vi "get limits from circle.vi"(8 "Radius":dbl, 10 "Current Location":T1 {"Position"."Position Y" format="%#.3f"; "Position"."Position X" format="%#.3f"}, 11 "Center location":T1 {"Position"."Position Y" format="%#.3f"; "Position"."Position X" format="%#.3f"}) -> (0 "Ymax given x":dbl, 1 "Ymin given x":dbl, 2 "Xmax given y":dbl, 3 "Xmin given y":dbl)   [LabVIEW 2017]
uses:
  location.ctl
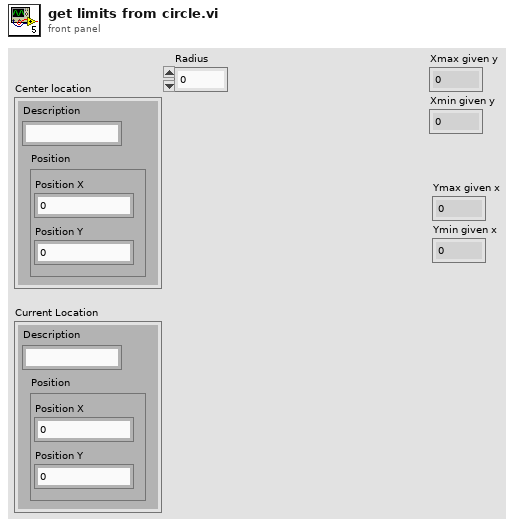
[diagram p1: front panel]
types:
  T1 = typedef "location.ctl" = cluster{"Description":string, "Position":cluster{"Position X":dbl, "Position Y":dbl}}
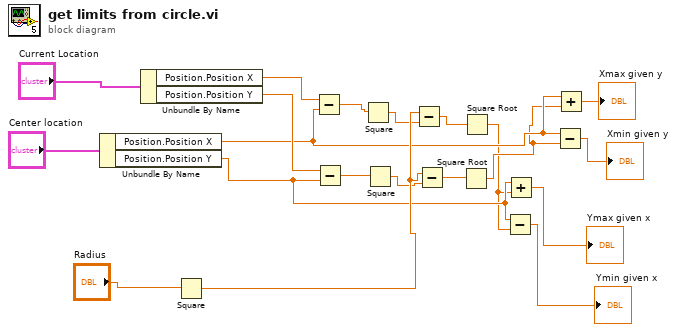
[diagram p0: block diagram]
diagram:
  n1 = Unbundle By Name("Center location") -> ("Position.Position X"=w6:dbl, "Position.Position Y"=w4:dbl)
  n2 = Unbundle By Name("Current Location") -> ("Position.Position X"=w18:dbl, "Position.Position Y"=w17:dbl)
  n3 = Square(x="Radius") -> (x^2=w13:dbl)
  n4 = Subtract(x=w18, y=w6) -> (x-y=w15:dbl)
  n5 = Subtract(x=w17, y=w4) -> (x-y=w14:dbl)
  n6 = Square(x=w15) -> (x^2=w12:dbl)
  n7 = Square(x=w14) -> (x^2=w11:dbl)
  n8 = Subtract(x=w13, y=w12) -> (x-y=w10:dbl)
  n9 = Subtract(x=w13, y=w11) -> (x-y=w9:dbl)
  n10 = Square Root(x=w9) -> (sqrt(x)=w5:dbl)
  n11 = Square Root(x=w10) -> (sqrt(x)=w3:dbl)
  n12 = Subtract(x=w4, y=w3) -> (x-y=→"Ymin given x":dbl)
  n13 = Add(x=w4, y=w3) -> (x+y=→"Ymax given x":dbl)
  n14 = Subtract(x=w6, y=w5) -> (x-y=→"Xmin given y":dbl)
  n15 = Add(x=w6, y=w5) -> (x+y=→"Xmax given y":dbl)
